vi "Practica 5.vi"() -> ()   [LabVIEW 2020]
panel:
  out "Impar":bool
  out "Par":bool
  in  "Numero":dbl
  out "Decimal":i16
  in  "2^3":bool
  in  "2^2":bool
  in  "2^1":bool
  in  "2^0":bool
  out "NAND":bool
  out "XOR":bool
  in  "Y 2":bool
  in  "X 2":bool
  in  "B 2":bool
  in  "A 2":bool
  out "OR":bool
  out "AND":bool
  in  "Y":bool
  in  "X":bool
  in  "B":bool
  in  "A":bool
  out "Rad 1":dbl
  in  "Grados 1":dbl
  out "F°":dbl
  out "Grados":dbl
  in  "Rad":dbl
  in  "C°":dbl
  # "COMPUERTAS"
  # "Conversión"
  # "Binario a Decimal"
  # "DETECTOR"
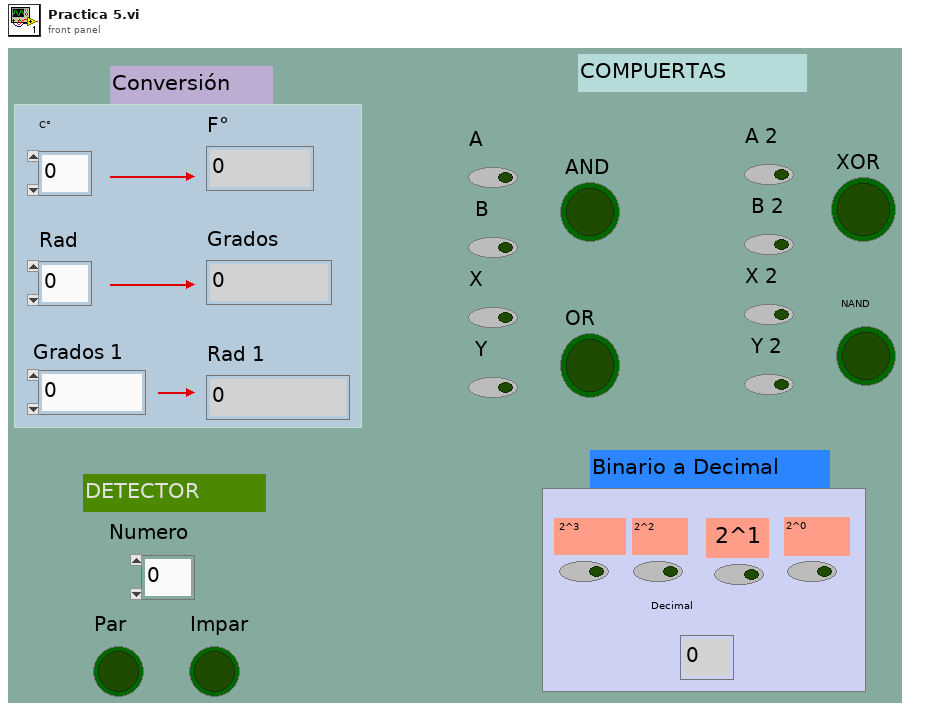
[diagram p1: front panel]
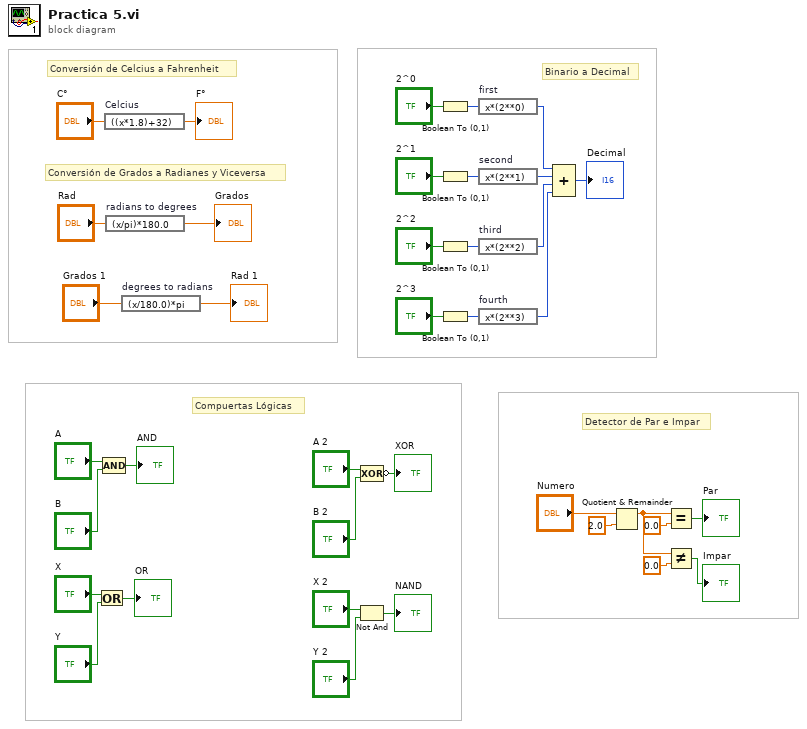
[diagram p0: block diagram]
diagram:
  # "Detector de Par e Impar"
  # "Compuertas Lógicas"
  # "Conversión de Celcius a Fahrenheit"
  # "Conversión de Grados a Radianes y Viceversa"
  # "Binario a Decimal"
  n1 = Or(x="X", y="Y") -> (x .or. y?=→"OR":bool)
  n2 = Compound Arithmetic op=AND("A", "B") -> (→"AND":bool)
  n3 = expression code="((x*1.8)+32)" "Celcius"("C°") -> (→"F°":dbl)
  n4 = expression code="(x/pi)*180.0" "radians to degrees"("Rad") -> (→"Grados":dbl)
  n5 = expression code="(x/180.0)*pi" "degrees to radians"("Grados 1") -> (→"Rad 1":dbl)
  n6 = Not And(1:"Y 2", 2:"X 2") -> (0:→"NAND":bool)
  n7 = Compound Arithmetic op=XOR("A 2", "B 2") -> (invert →"XOR":bool)
  n8 = Boolean To (0,1)(Boolean="2^0") -> (0, 1=w15:i16)
  n9 = Boolean To (0,1)(Boolean="2^1") -> (0, 1=w13:i16)
  n10 = Boolean To (0,1)(Boolean="2^2") -> (0, 1=w12:i16)
  n11 = Boolean To (0,1)(Boolean="2^3") -> (0, 1=w11:i16)
  n12 = expression code="x*(2**0)" "first"(w15) -> (w14:i16)
  n13 = expression code="x*(2**1)" "second"(w13) -> (w10:i16)
  n14 = expression code="x*(2**2)" "third"(w12) -> (w9:i16)
  n15 = expression code="x*(2**3)" "fourth"(w11) -> (w8:i16)
  n16 = Compound Arithmetic op=ADD(w14, w10, w9, w8) -> (→"Decimal":i16)
  n17 = Quotient & Remainder(x="Numero", y=2.0) -> (x-y*floor(x/y)=w3:dbl)  [unwired: 1 out]
  n18 = Equal?(x=w3, y=0.0) -> (x = y?=→"Par":bool)
  n19 = Not Equal?(x=w3, y=0.0) -> (x != y?=→"Impar":bool)
